vi "EnumApplications.vi"(8 "error in (no error)":errorcluster) -> (0 "error out":errorcluster, 2 "Application Names":string[](array[string]), 3 "Application References":refnum<vi>[](array[refnum]))   [LabVIEW 2020]
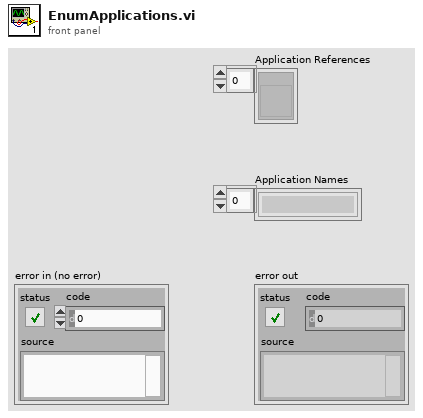
[diagram p1: front panel]
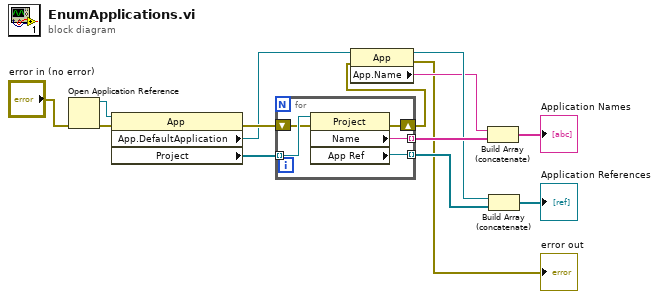
[diagram p0: block diagram]
diagram:
  n1 = Open Application Reference(8:"error in (no error)") -> (0:w14:errorcluster, 3:w13:refnum<vi>)  [unwired: 3 in]
  n2 = property class="App"(reference=w13, error in=w14) -> (error out=w10:errorcluster, "App.DefaultApplication"=w6:refnum<vi>, "Project"=w3:refnum<vi>[])  [unwired: 1 out]
  n3 = for {
    tunnel: w3 -> [w19] mode=indexing
    tunnel: [w15] -> w12 mode=indexing
    shift-right: [w17] -> w2
    shift-left: w10 -> [w18]
    tunnel: [w16] -> w8 mode=indexing
    n4 = property class="Project"(reference=w19, error in=w18) -> (error out=w17:errorcluster, "Name"=w16:string, "App Ref"=w15:refnum<vi>)  [unwired: 1 out]
  }
  n5 = property class="App"(reference=w6, error in=w2) -> (reference out=w5:refnum<vi>, error out=→"error out":errorcluster, "App.Name"=w4:string)
  n6 = Build Array (concatenate)(w4, w8) -> (→"Application Names":string[])
  n7 = Build Array (concatenate)(w5, w12) -> (→"Application References":refnum<vi>[])
